vi "Dubble_Butterwidth_Filter.vi"(1 "Higher Cut-Off":dbl, 2 "sampling freq: fs":dbl=1.0 format="%0.2f", 3 "Array in":dbl[][](array[numeric]), 4 "filter type":T1) -> (0 "Array out":dbl[][](array[numeric]))   [LabVIEW 2023]
uses:
  <vilib>/Analysis/3filter.llb/Filter Passband Type.ctl
  <vilib>/Analysis/3filter.llb/Butterworth Filter (DBL).vi
  <vilib>/Analysis/NI_AALBase.lvlib
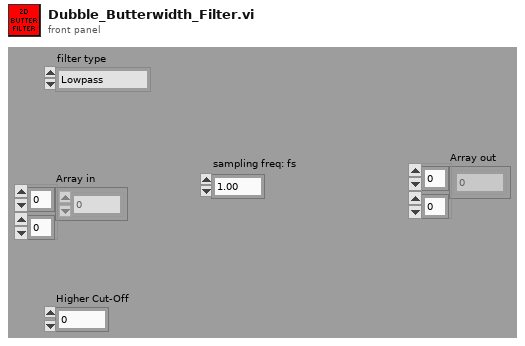
[diagram p1: front panel]
types:
  T1 = typedef "NI_AALBase.lvlib/Filter Passband Type.ctl" = enum32{"Lowpass", "Highpass", "Bandpass", "Bandstop"}
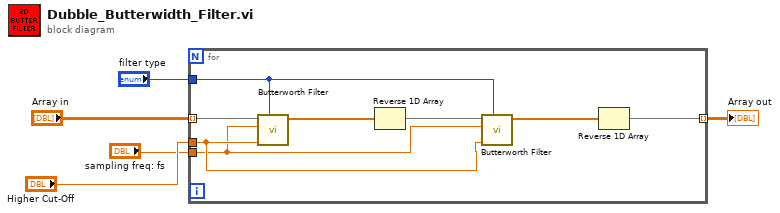
[diagram p0: block diagram]
diagram:
  n1 = for {
    tunnel: "Array in" -> [w11] mode=indexing
    tunnel: [w9] -> w4 mode=indexing
    tunnel: "Higher Cut-Off" -> [w7]
    tunnel: "filter type" -> [w8]
    tunnel: "sampling freq: fs" -> [w6]
    n2 = call-poly <vilib>:"Butterworth Filter.vi"("filter type"=w8, "low cutoff freq: fl"=w7, "sampling freq: fs"=w6, "X"=w11) -> ("Filtered X"=w12:dbl[])  [unwired: 4 in, 1 out]
    n3 = Reverse 1D Array(array=w12) -> (reversed array=w13:dbl[])
    n4 = call-poly <vilib>:"Butterworth Filter.vi"("filter type"=w8, "low cutoff freq: fl"=w7, "sampling freq: fs"=w6, "X"=w13) -> ("Filtered X"=w10:dbl[])  [unwired: 4 in, 1 out]
    n5 = Reverse 1D Array(array=w10) -> (reversed array=w9:dbl[])
  }
  "Array out" <- w4
